vi "shiftDelayState.vi"(8 "u(k)":sgl, 9 "Xd_in":T1=[0.0, 0.0, 0.0, 0.0, 0.0, 0.0, 0.0, 0.0, 0.0, 0.0, 0.0, 0.0] caption="Xd_In", 11 "Nd":u8) -> (1 "Xd_out":T1, 3 "yd=C*Xd(k)":sgl)   [LabVIEW 2017]
uses:
  controls/Xdelay.ctl
  <vilib>/Platform/TimedLoop/XDataNode/timing_clust.ctl
  <vilib>/Platform/TimedLoop/XDataNode/nitl_modes.ctl
  <vilib>/Platform/TimedLoop/XDataNode/wakeup.ctl
  <vilib>/rvi/Emulation/niFpgaSctlEmulationGetInTimedLoop.vi
  <vilib>/rvi/Emulation/niFpgaEmulationReportErrorSimple.vi
  <vilib>/rvi/Emulation/niFpgaGetClockAttributes.vi
  <vilib>/rvi/Emulation/niFpgaCriticalErrorInLSC.vi
  <vilib>/Platform/TimedLoop/XDataNode/XDataNode.xnode
  <vilib>/Platform/TimedLoop/XDataNode/XDNodeRunTimeDep.lvlib
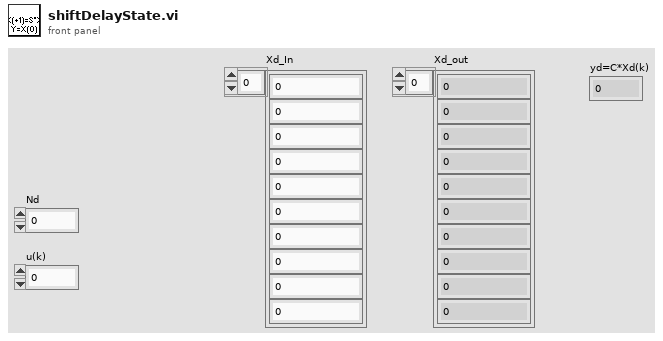
[diagram p1: front panel]
types:
  T1 = typedef "Xdelay.ctl" = sgl[]
  T2 = typedef "XDNodeRunTimeDep.lvlib/timing_clust.ctl" = cluster{"Expected End [f-1]":u64, "Actual End [f-1]":u64, "Finished Late? [f-1]":bool, "Expected End [i-1]":u64, "Actual End [i-1]":u64, "Finished Late? [i-1]":bool, "Expected Start [i]":u64, "Actual Start [i]":u64, "Expected Start [f]":u64, "Actual Start [f]":u64, "Source Name":string, "Structure Name":string, "Period":i64, "Deadline":i64, "Offset":i64, "Start":i64, "Priority":i32, "Timeout":i32, "Mode":T3, "Wakeup Reason":T4, "Error":errorcluster, "Source Type":string, "Secondary Source Type":string, "Global End Time":u64, "Global Start Time":u64, "Frame Duration":u64, "Iteration Duration":u64, "Assigned CPU":i32, "I/O Scan Engine Mode":u32}
  T3 = typedef "XDNodeRunTimeDep.lvlib/nitl_modes.ctl" = enum32{"No Change", "Process missed periods, maintain original phase", "Discard missed periods, maintain original phase", "Process missed periods, ignore original phase", "Discard missed periods, ignore original phase"}
  T4 = typedef "XDNodeRunTimeDep.lvlib/wakeup.ctl" = enum32{"Normal", "Aborted", "Asynchronous wakeup", "Timing source error", "Timed loop error", "Timeout"}
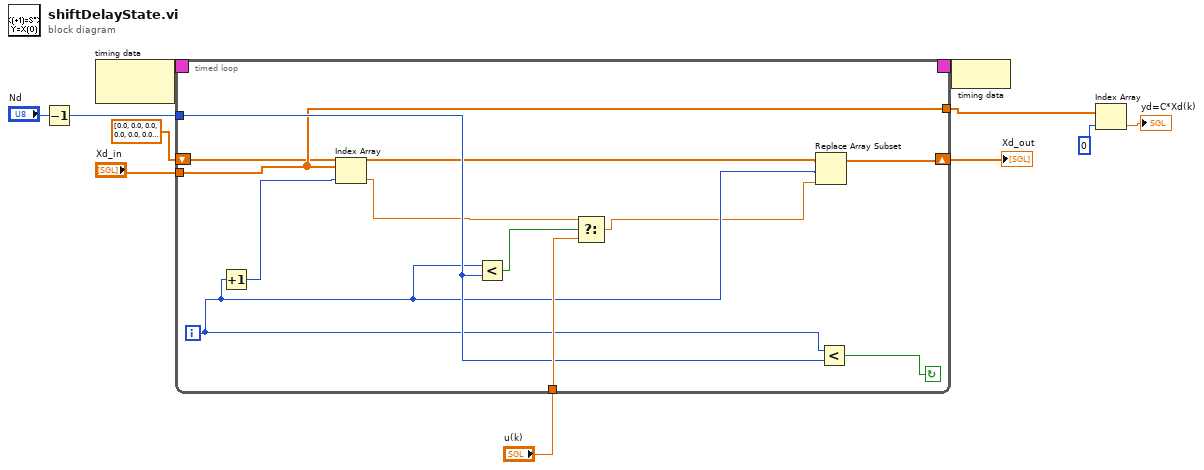
[diagram p0: block diagram]
diagram:
  n1 = Decrement(x="Nd") -> (x-1=w7:u8)
  n2 = node-c288() -> (w11:T2)  [unwired: 1 in]
  n3 = timed-loop {
    tunnel: w7 -> [w19]
    timing: w11 -> [_]
    timing-out: [_] -> w10
    tunnel: "u(k)" -> [w22]
    tunnel: "Xd_in" -> [w16]
    shift-right: [w15] -> w3
    shift-left: sgl[] [0.0, 0.0, 0.0, 0.0, 0.0, 0.0, 0.0, 0.0, 0.0, 0.0, 0.0, 0.0] ("Xd_in 2") -> [w14]
    tunnel: [w16] -> w1
    i -> [w13]
    stop <- w20 continue-if-true
    n4 = Increment(x=w13) -> (x+1=w18:i32)
    n5 = Index Array(array=w16, index=w18) -> (element=w17:sgl)
    n6 = Less?(x=w13, y=w19) -> (x < y?=w21:bool)
    n7 = Select(t=w17, s=w21, f=w22) -> (s? t:f=w12:sgl)
    n8 = Replace Array Subset(array=w14, new element=w12, index=w13) -> (w15:sgl[])
    n9 = Less?(x=w13, y=w19) -> (x < y?=w20:bool)
  }
  "Xd_out" <- w3
  n10 = node-c288(w10) -> ()
  n11 = Index Array(array=w1, index=i16 0) -> (element=→"yd=C*Xd(k)":sgl)
